vi "SR430_read_ascdata.vi"(0 "address":T1, 5 "error in (no error)":errorcluster) -> (14 "address out":T1, 16 "Data":dbl[](array[numeric]) format="%.2f", 17 "dataSum":dbl format="%.2f", 19 "error out":errorcluster)   [LabVIEW 2015, in "SR430Driver.lvlib"]
doc: "Reads the entire display memory data record in ascii format. \n\nCopyright (C)\nGesellschaft für Schwerionenforschung, GSI\nPlanckstr. 1\n64291 Darmstadt\nGermany\n\nContact: D.Beck@gsi.de \n\nThis program is free software; you can redistribute it and/or modify it under the terms of the \nGNU General Public License as published by the Free Software Foundation; either version 2 of the license, or (at your option) any later version.\n\nThis program is distributed in the hope that it will be useful, but WITHOUT ANY WARRANTY; without even the implied warranty of MERCHANTABILITY or FITNESS FOR A PARTICULAR PURPOSE. See the GNU General License for more details (http://www.gnu.org).\n\nGesellschaft für Schwerionenforschung, GSI\nPlanckstr. 1, 64291 Darmstadt, Germany\nFor all questions and ideas contact: M.Richter@gsi.de, K.Poppensieker, H.Brand@gsi.de or D.Beck@gsi.de.\nLast update: 11-APR-2002"
uses:
  SR430Driver.lvlib
  SR430_VISA Control.ctl
panel:
  # "SR430 Read ASCII Data"
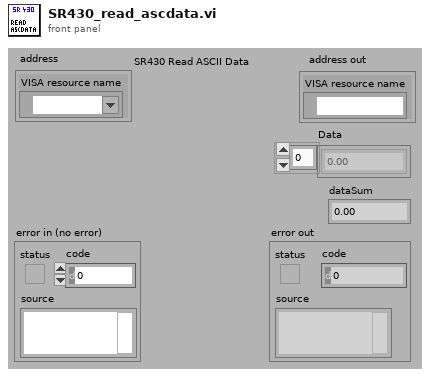
[diagram p1: front panel]
types:
  T1 = typedef "SR430Driver.lvlib/SR430_VISA Control.ctl" = cluster{"VISA resource name":refnum<visa-resource-name>}
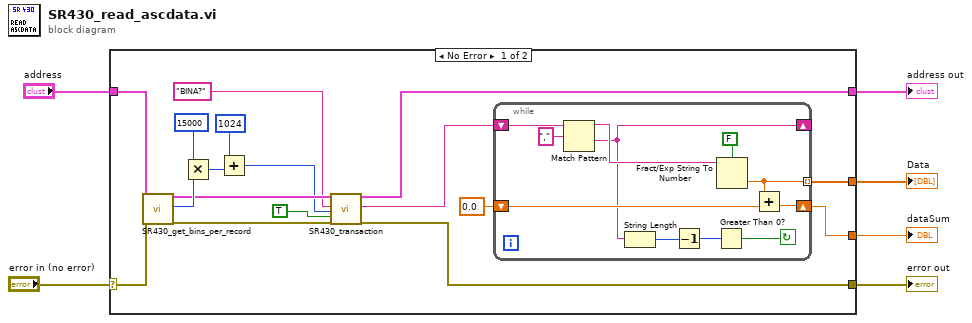
[diagram p0: block diagram]
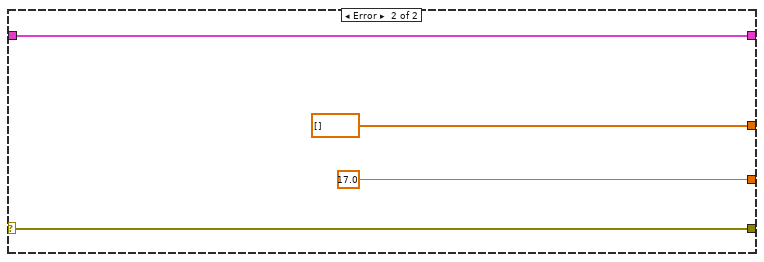
[diagram p2: hidden frame]
diagram:
  n1 = case shown="No Error" "error in (no error)" {
    selector: "error in (no error)" -> [w22 w36]
    tunnel: [w19 dbl[] []] -> w1
    tunnel: "address" -> [w20 w35]
    tunnel: [w7 w36] -> w6
    tunnel: [w17 17.0] -> w4
    tunnel: [w9 w35] -> w2
    frame No Error {
      n2 = call "SR430_get_bins_per_record.vi"("address"=w20, "error in (no error)"=w22) -> ("address out"=w14:T1, "binsPerRecord"=w21:i32, "error out"=w11:errorcluster)  [unwired: 15 in]
      n3 = Multiply(x=15000 ("byte count"), y=w21) -> (x*y=w16:i32)
      n4 = Add(x=1024, y=w16) -> (x+y=w13:i32)
      n5 = call "SR430_transaction.vi"("SR430 VISA Cluster"=w14, "SR430 Command String"="BINA?" ("write buffer"), "Bytes to read (1024)"=w13, "Read (FALSE)"=TRUE, "error in (no error)"=w11) -> ("dup SR430 VISA Cluster"=w9:T1, "SR430 Response"=w8:string, "error out"=w7:errorcluster)  [unwired: 11 in, 1 out]
      n6 = while {
        shift-left: 0.0 -> [w32]
        shift-right: [w29] -> w17
        tunnel: [w30] -> w19 mode=indexing
        shift-left: w8 -> [w28]
        shift-right: [w27] -> _
        stop <- w31 continue-if-true
        n7 = Match Pattern(string=w28, regular expression=",") -> (before substring=w33:string, after substring=w27:string)  [unwired: 1 in, 2 out]
        n8 = String Length(string=w27) -> (length=w26:i32)
        n9 = Decrement(x=w26) -> (x-1=w25:i32)
        n10 = Greater Than 0?(x=w25) -> (x > 0?=w31:bool)
        n11 = Fract/Exp String To Number(use system decimal point (T)=FALSE, string=w33) -> (number=w30:dbl)  [unwired: 2 in, 1 out]
        n12 = Add(x=w30, y=w32) -> (x+y=w29:dbl)
      }
    }
    frame Error {
    }
  }
  "error out" <- w6
  "Data" <- w1
  "dataSum" <- w4
  "address out" <- w2
